vi "Get.vi"(8 "error in (no error)":errorcluster, 11 "Waveform Generator in":refnum<class "Waveform Generator.lvclass">) -> (0 "error out":errorcluster, 2 "Value":dbl, 3 "Waveform Generator out":refnum<class "Waveform Generator.lvclass">)   [LabVIEW 2015, in "Waveform Generator.lvclass"]
uses:
  Waveform Generator.lvclass
  Waveform Generator.lvclass/Waveform Generator.ctl
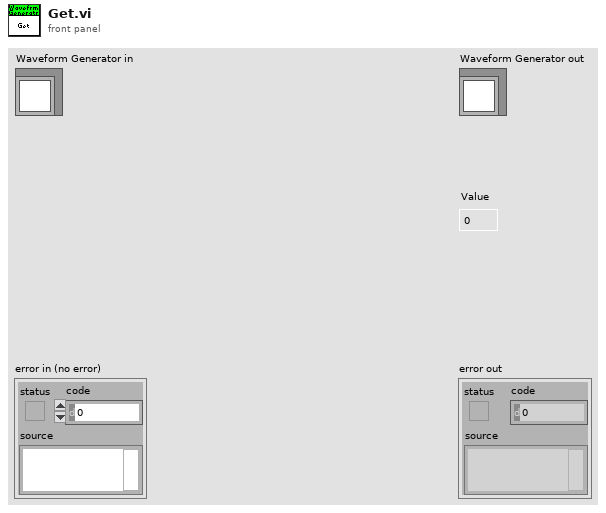
[diagram p1: front panel]
types:
  T1 = typedef "FAMT Typedefs.lvlib/Waveform Types.ctl" = enum16{"Sine", "Triangle", "Square", "Sawtooth", "Chirp", "Gaussian", "Trapezoid"}
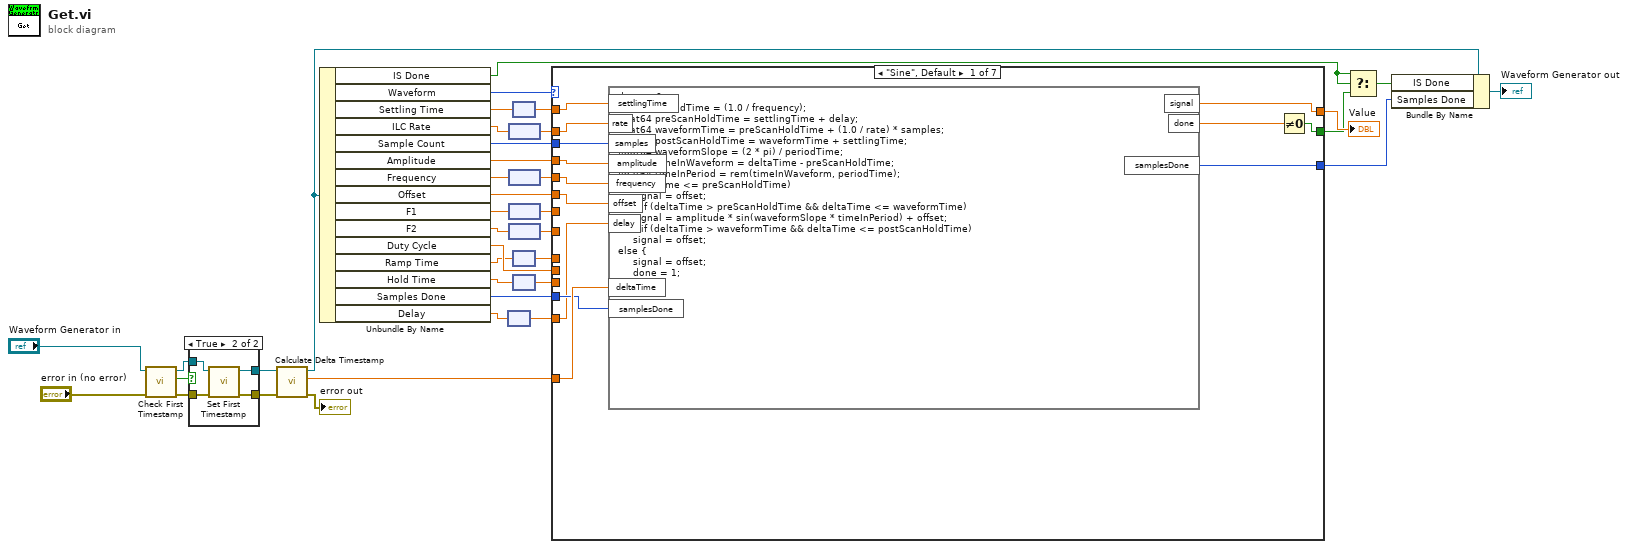
[diagram p0: block diagram]
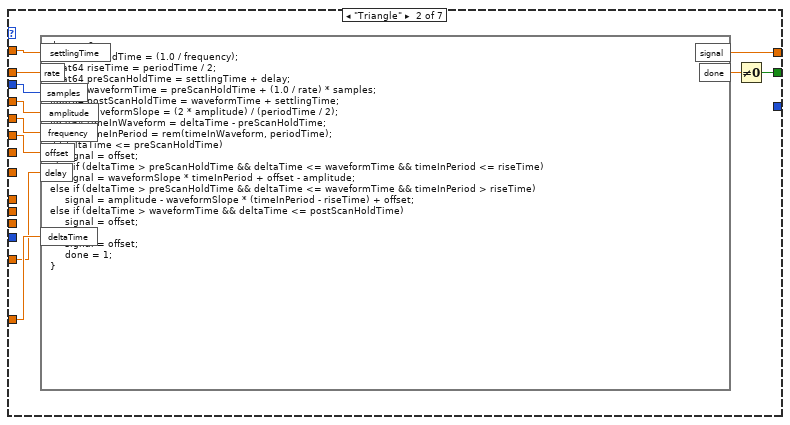
[diagram p2: hidden frame]
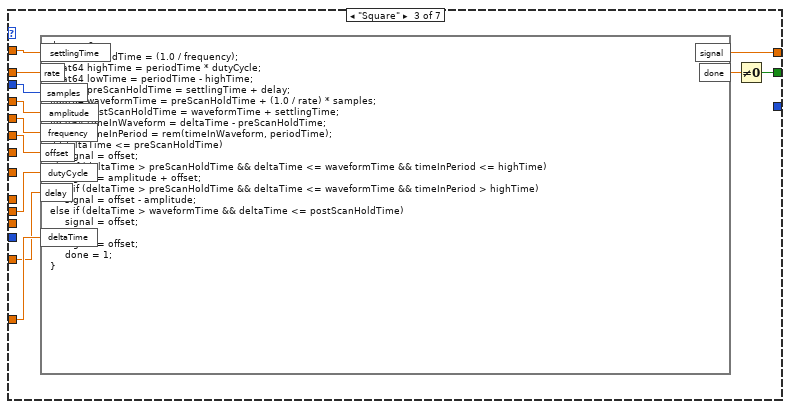
[diagram p3: hidden frame]
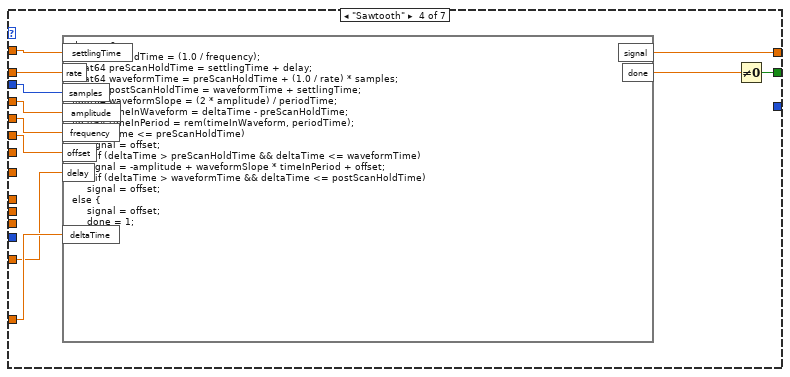
[diagram p4: hidden frame]
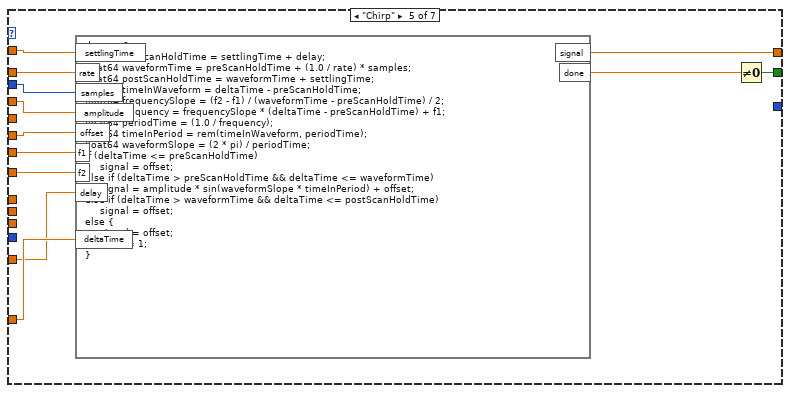
[diagram p5: hidden frame]
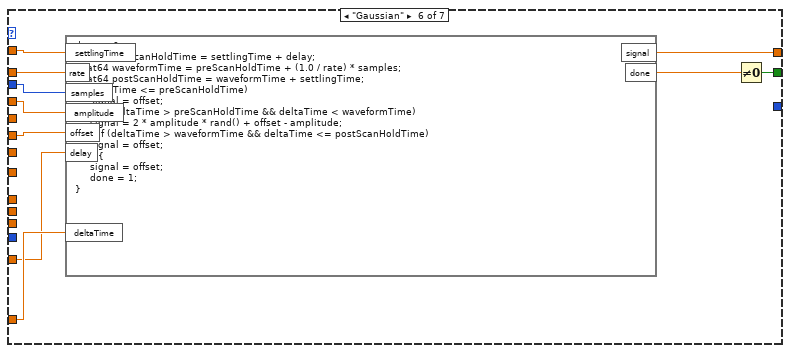
[diagram p6: hidden frame]
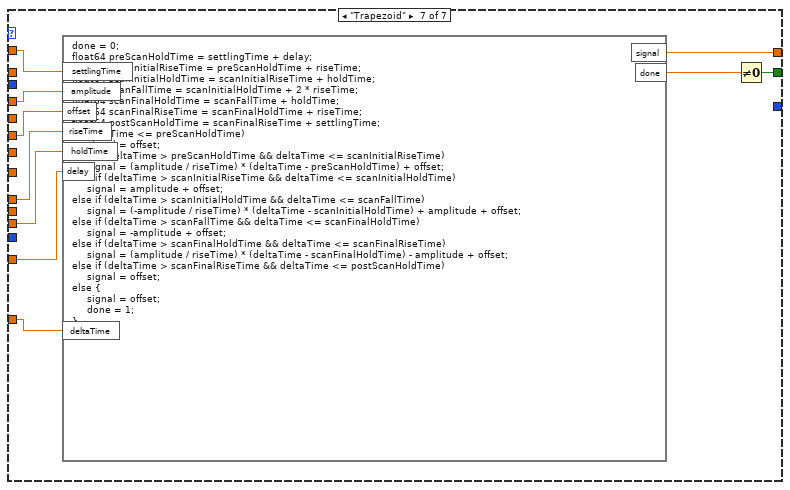
[diagram p7: hidden frame]
diagram:
  n1 = call "Check First Timestamp.vi"("error in (no error)"="error in (no error)", "Waveform Generator in"="Waveform Generator in") -> ("error out"=w36:errorcluster, "Is First"=w38:bool, "Waveform Generator out"=w37:refnum<class "Waveform Generator.lvclass">)  [unwired: 7 in]
  n2 = case shown="True" w38 {
    tunnel: w37 -> [w40 w44]
    tunnel: [w40 w43] -> w35
    tunnel: w36 -> [w39 w42]
    tunnel: [w39 w41] -> w34
    frame False {
    }
    frame True {
      n3 = call "Set First Timestamp.vi"("error in (no error)"=w42, "Waveform Generator in"=w44) -> ("error out"=w41:errorcluster, "Waveform Generator out"=w43:refnum<class "Waveform Generator.lvclass">)  [unwired: 8 in]
    }
  }
  n4 = call "Calculate Delta Timestamp.vi"("error in (no error)"=w34, "Waveform Generator in"=w35) -> ("error out"=→"error out":errorcluster, "Delta Timestamp"=w21:dbl, "Waveform Generator out"=w11:refnum<class "Waveform Generator.lvclass">)  [unwired: 7 in]
  n5 = Unbundle By Name(w11) -> ("IS Done"=w8:bool, "Waveform"=w19:T1, "Settling Time"=w32:dbl[unit], "ILC Rate"=w30:dbl[unit], "Sample Count"=w29:u32, "Amplitude"=w4:dbl, "Frequency"=w18:dbl[unit], "Offset"=w3:dbl, "F1"=w27:dbl[unit], "F2"=w25:dbl[unit], "Duty Cycle"=w16:dbl, "Ramp Time"=w15:dbl[unit], "Hold Time"=w14:dbl[unit], "Samples Done"=w5:u32, "Delay"=w2:dbl[unit])
  n6 = node(w2) -> (w1:dbl)
  n7 = node(w30) -> (w28:dbl)
  n8 = node(w18) -> (w17:dbl)
  n9 = node(w27) -> (w26:dbl)
  n10 = node(w25) -> (w24:dbl)
  n11 = node(w32) -> (w31:dbl)
  n12 = node(w15) -> (w12:dbl)
  n13 = node(w14) -> (w13:dbl)
  n14 = case shown="\"Sine\", Default" w19 {
    tunnel: [w50 w68 w72 w84 w95 w108 w117] -> w33
    tunnel: w31 -> [w57 w61 w74 w91 w96 w113 w123]
    tunnel: w29 -> [w55 w63 w76 w89 w98 w111 _]
    tunnel: w28 -> [w56 w62 w75 w90 w97 w112 _]
    tunnel: w4 -> [w54 w64 w77 w88 w99 w110 w122]
    tunnel: w3 -> [w53 w66 w79 w86 w100 w105 w121]
    tunnel: w26 -> [_ _ _ _ w101 _ _]
    tunnel: w24 -> [_ _ _ _ w102 _ _]
    tunnel: w21 -> [w51 w67 w73 w85 w103 w109 w118]
    tunnel: w17 -> [w52 w65 w78 w87 _ _ _]
    tunnel: w16 -> [_ _ w80 _ _ _ _]
    tunnel: w13 -> [_ _ _ _ _ _ w120]
    tunnel: w12 -> [_ _ _ _ _ _ w119]
    tunnel: [w49 w59 w71 w82 w93 w106 w115] -> w9
    tunnel: [w47 _ _ _ _ _ _] -> w6
    tunnel: w5 -> [w46 _ _ _ _ _ _]
    tunnel: w1 -> [w45 w58 w69 w81 w92 w104 w114]
    frame "Sine", Default {
      n15 = formula code="done = 0;\nfloat64 periodTime = (1.0 / frequency);\nfloat64 preScanHoldTime = settlingTime + delay;\nfloat64 waveformTime = preScanHoldTime + (1.0 / rate) * samples;\nfloat64 postScanHoldTime = waveformTime + settlingTime;\nfloat64 waveformSlope = (2 * pi) / periodTime;\nfloat64 timeInWaveform = deltaTime - preScanHoldTime;\nfloat64 timeInPeriod = rem(timeInWaveform, periodTime);\nif (deltaTime <= preScanHoldTime)\n     signal = offset;\nelse if (deltaTime > preScanHoldTime && deltaTime <= waveformTime)\n     signal = amplitude * sin(waveformSlope * timeInPeriod) + offset;\nelse if (deltaTime > waveformTime && deltaTime <= postScanHoldTime)\n     signal = offset;\nelse {\n     signal = offset;\n     done = 1;\n}"("rate"=w56, "settlingTime"=w57, "samples"=w55, "amplitude"=w54, "frequency"=w52, "offset"=w53, "deltaTime"=w51, "samplesDone"=w46, "delay"=w45) -> ("signal"=w50:dbl, "done"=w48:dbl, "samplesDone"=w47:u32)
      n16 = Not Equal To 0?(x=w48) -> (x != 0?=w49:bool)
    }
    frame "Triangle" {
      n17 = formula code="done = 0;\nfloat64 periodTime = (1.0 / frequency);\nfloat64 riseTime = periodTime / 2;\nfloat64 preScanHoldTime = settlingTime + delay;\nfloat64 waveformTime = preScanHoldTime + (1.0 / rate) * samples;\nfloat64 postScanHoldTime = waveformTime + settlingTime;\nfloat64 waveformSlope = (2 * amplitude) / (periodTime / 2);\nfloat64 timeInWaveform = deltaTime - preScanHoldTime;\nfloat64 timeInPeriod = rem(timeInWaveform, periodTime);\nif (deltaTime <= preScanHoldTime)\n     signal = offset;\nelse if (deltaTime > preScanHoldTime && deltaTime <= waveformTime && timeInPeriod <= riseTime)\n     signal = waveformSlope * timeInPeriod + offset - amplitude;\nelse if (deltaTime > preScanHoldTime && deltaTime <= waveformTime && timeInPeriod > riseTime)\n     signal = amplitude - waveformSlope * (timeInPeriod - riseTime) + offset;\nelse if (deltaTime > waveformTime && deltaTime <= postScanHoldTime)\n     signal = offset;\nelse {\n     signal = offset;\n     done = 1;\n}"("rate"=w62, "settlingTime"=w61, "samples"=w63, "amplitude"=w64, "frequency"=w65, "offset"=w66, "deltaTime"=w67, "delay"=w58) -> ("signal"=w68:dbl, "done"=w60:dbl)
      n18 = Not Equal To 0?(x=w60) -> (x != 0?=w59:bool)
    }
    frame "Square" {
      n19 = formula code="done = 0;\nfloat64 periodTime = (1.0 / frequency);\nfloat64 highTime = periodTime * dutyCycle;\nfloat64 lowTime = periodTime - highTime;\nfloat64 preScanHoldTime = settlingTime + delay;\nfloat64 waveformTime = preScanHoldTime + (1.0 / rate) * samples;\nfloat64 postScanHoldTime = waveformTime + settlingTime;\nfloat64 timeInWaveform = deltaTime - preScanHoldTime;\nfloat64 timeInPeriod = rem(timeInWaveform, periodTime);\nif (deltaTime <= preScanHoldTime)\n     signal = offset;\nelse if (deltaTime > preScanHoldTime && deltaTime <= waveformTime && timeInPeriod <= highTime)\n     signal = amplitude + offset;\nelse if (deltaTime > preScanHoldTime && deltaTime <= waveformTime && timeInPeriod > highTime)\n     signal = offset - amplitude;\nelse if (deltaTime > waveformTime && deltaTime <= postScanHoldTime)\n     signal = offset;\nelse {\n     signal = offset;\n     done = 1;\n}"("rate"=w75, "settlingTime"=w74, "samples"=w76, "amplitude"=w77, "frequency"=w78, "offset"=w79, "deltaTime"=w73, "dutyCycle"=w80, "delay"=w69) -> ("signal"=w72:dbl, "done"=w70:dbl)
      n20 = Not Equal To 0?(x=w70) -> (x != 0?=w71:bool)
    }
    frame "Sawtooth" {
      n21 = formula code="done = 0;\nfloat64 periodTime = (1.0 / frequency);\nfloat64 preScanHoldTime = settlingTime + delay;\nfloat64 waveformTime = preScanHoldTime + (1.0 / rate) * samples;\nfloat64 postScanHoldTime = waveformTime + settlingTime;\nfloat64 waveformSlope = (2 * amplitude) / periodTime;\nfloat64 timeInWaveform = deltaTime - preScanHoldTime;\nfloat64 timeInPeriod = rem(timeInWaveform, periodTime);\nif (deltaTime <= preScanHoldTime)\n     signal = offset;\nelse if (deltaTime > preScanHoldTime && deltaTime <= waveformTime)\n     signal = -amplitude + waveformSlope * timeInPeriod + offset;\nelse if (deltaTime > waveformTime && deltaTime <= postScanHoldTime)\n     signal = offset;\nelse {\n     signal = offset;\n     done = 1;\n}"("rate"=w90, "settlingTime"=w91, "samples"=w89, "amplitude"=w88, "frequency"=w87, "offset"=w86, "deltaTime"=w85, "delay"=w81) -> ("signal"=w84:dbl, "done"=w83:dbl)
      n22 = Not Equal To 0?(x=w83) -> (x != 0?=w82:bool)
    }
    frame "Chirp" {
      n23 = formula code="done = 0;\nfloat64 preScanHoldTime = settlingTime + delay;\nfloat64 waveformTime = preScanHoldTime + (1.0 / rate) * samples;\nfloat64 postScanHoldTime = waveformTime + settlingTime;\nfloat64 timeInWaveform = deltaTime - preScanHoldTime;\nfloat64 frequencySlope = (f2 - f1) / (waveformTime - preScanHoldTime) / 2;\nfloat64 frequency = frequencySlope * (deltaTime - preScanHoldTime) + f1;\nfloat64 periodTime = (1.0 / frequency);\nfloat64 timeInPeriod = rem(timeInWaveform, periodTime);\nfloat64 waveformSlope = (2 * pi) / periodTime;\nif (deltaTime <= preScanHoldTime)\n     signal = offset;\nelse if (deltaTime > preScanHoldTime && deltaTime <= waveformTime)\n     signal = amplitude * sin(waveformSlope * timeInPeriod) + offset;\nelse if (deltaTime > waveformTime && deltaTime <= postScanHoldTime)\n     signal = offset;\nelse {\n     signal = offset;\n     done = 1;\n}"("rate"=w97, "settlingTime"=w96, "samples"=w98, "amplitude"=w99, "offset"=w100, "deltaTime"=w103, "f1"=w101, "f2"=w102, "delay"=w92) -> ("signal"=w95:dbl, "done"=w94:dbl)
      n24 = Not Equal To 0?(x=w94) -> (x != 0?=w93:bool)
    }
    frame "Gaussian" {
      n25 = formula code="done = 0;\nfloat64 preScanHoldTime = settlingTime + delay;\nfloat64 waveformTime = preScanHoldTime + (1.0 / rate) * samples;\nfloat64 postScanHoldTime = waveformTime + settlingTime;\nif (deltaTime <= preScanHoldTime)\n     signal = offset;\nelse if (deltaTime > preScanHoldTime && deltaTime < waveformTime)\n     signal = 2 * amplitude * rand() + offset - amplitude;\nelse if (deltaTime > waveformTime && deltaTime <= postScanHoldTime)\n     signal = offset;\nelse {\n     signal = offset;\n     done = 1;\n}"("settlingTime"=w113, "amplitude"=w110, "offset"=w105, "deltaTime"=w109, "rate"=w112, "samples"=w111, "delay"=w104) -> ("signal"=w108:dbl, "done"=w107:dbl)
      n26 = Not Equal To 0?(x=w107) -> (x != 0?=w106:bool)
    }
    frame "Trapezoid" {
      n27 = formula code="done = 0;\nfloat64 preScanHoldTime = settlingTime + delay;\nfloat64 scanInitialRiseTime = preScanHoldTime + riseTime;\nfloat64 scanInitialHoldTime = scanInitialRiseTime + holdTime;\nfloat64 scanFallTime = scanInitialHoldTime + 2 * riseTime;\nfloat64 scanFinalHoldTime = scanFallTime + holdTime;\nfloat64 scanFinalRiseTime = scanFinalHoldTime + riseTime;\nfloat64 postScanHoldTime = scanFinalRiseTime + settlingTime;\nif (deltaTime <= preScanHoldTime)\n     signal = offset;\nelse if (deltaTime > preScanHoldTime && deltaTime <= scanInitialRiseTime)\n     signal = (amplitude / riseTime) * (deltaTime - preScanHoldTime) + offset;\nelse if (deltaTime > scanInitialRiseTime && deltaTime <= scanInitialHoldTime)\n     signal = amplitude + offset;\nelse if (deltaTime > scanInitialHoldTime && deltaTime <= scanFallTime)\n     signal = (-amplitude / riseTime) * (deltaTime - scanInitialHoldTime) + amplitude + offset;\nelse if (deltaTime > scanFallTime && deltaTime <= scanFinalHoldTime)\n     signal = -amplitude + offset;\nelse if (deltaTime > scanFinalHoldTime && deltaTime <= scanFinalRiseTime)\n     signal = (amplitude / riseTime) * (deltaTime - scanFinalHoldTime) - amplitude + offset;\nelse if (deltaTime > scanFinalRiseTime && deltaTime <= postScanHoldTime)\n     signal = offset;\nelse {\n     signal = offset;\n     done = 1;\n}"("deltaTime"=w118, "riseTime"=w119, "holdTime"=w120, "amplitude"=w122, "offset"=w121, "settlingTime"=w123, "delay"=w114) -> ("signal"=w117:dbl, "done"=w116:dbl)
      n28 = Not Equal To 0?(x=w116) -> (x != 0?=w115:bool)
    }
  }
  "Value" <- w33
  n29 = Select(t=w8, s=w8, f=w9) -> (s? t:f=w7:bool)
  n30 = Bundle By Name(cluster=w11, "IS Done"=w7, "Samples Done"=w6) -> (→"Waveform Generator out":refnum<class "Waveform Generator.lvclass">)
